vi "getPortAndIP.vi"(6 "error in (no error)":errorcluster, 7 "Device Name":string, 8 "This Vi":refnum<vi>) -> (0 "error out":errorcluster, 1 "Device Type":string, 2 "Remote Host":string="192.168.10.157", 3 "port or service name":u16=65400, 5 "reference out":refnum<vi>)   [LabVIEW 2020]
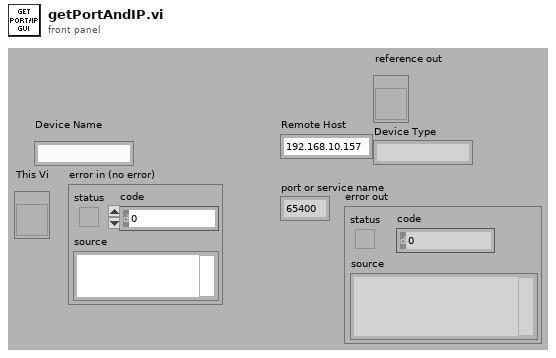
[diagram p1: front panel]
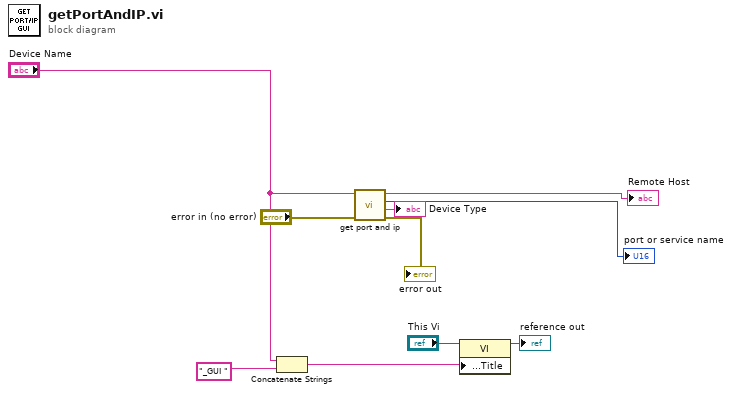
[diagram p0: block diagram]
diagram:
  n1 = Concatenate Strings("Device Name", "_GUI ") -> (w7:string)
  n2 = call "get port and ip.vi"("error in (no error)"="error in (no error)", "Device Name"="Device Name") -> ("error out"=→"error out":errorcluster, "Device Type"=→"Device Type":string, "remote port"=→"port or service name":u16, "remote host ip"=→"Remote Host":string)  [unwired: 6 in]
  n3 = property class="VI"(reference="This Vi", "Front Panel.Title"=w7) -> (reference out=→"reference out":refnum<vi>)  [unwired: 1 in, 1 out]
